vi "INIT R232 Seperate Mode.vi"(8 "error in (no error)":errorcluster, 11 "MC VISA resource in":refnum<visa-resource-name>="ASRL1::INSTR") -> (0 "MC error out":errorcluster, 1 "MC Init Complete":bool=TRUE, 3 "MC VISA resource  out":refnum<visa-resource-name>)   [LabVIEW 2009]
uses:
  <vilib>/Instr/_visa.llb/VISA Configure Serial Port (Instr).vi
panel:
  out "All Stop":bool
  out "Set Mode 3":bool
  in  "Mode command 3":string="^04 C0"
  out "Set Mode 2":bool
  in  "Mode command 2":string="^03 00"
  out "Set RS232 Control":bool
  out "Set Mode 1":bool
  in  "Mode command 1":string="^01 C4"
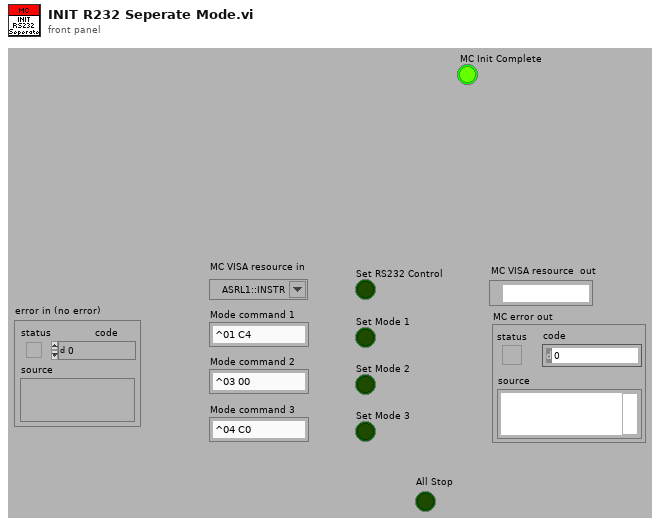
[diagram p1: front panel]
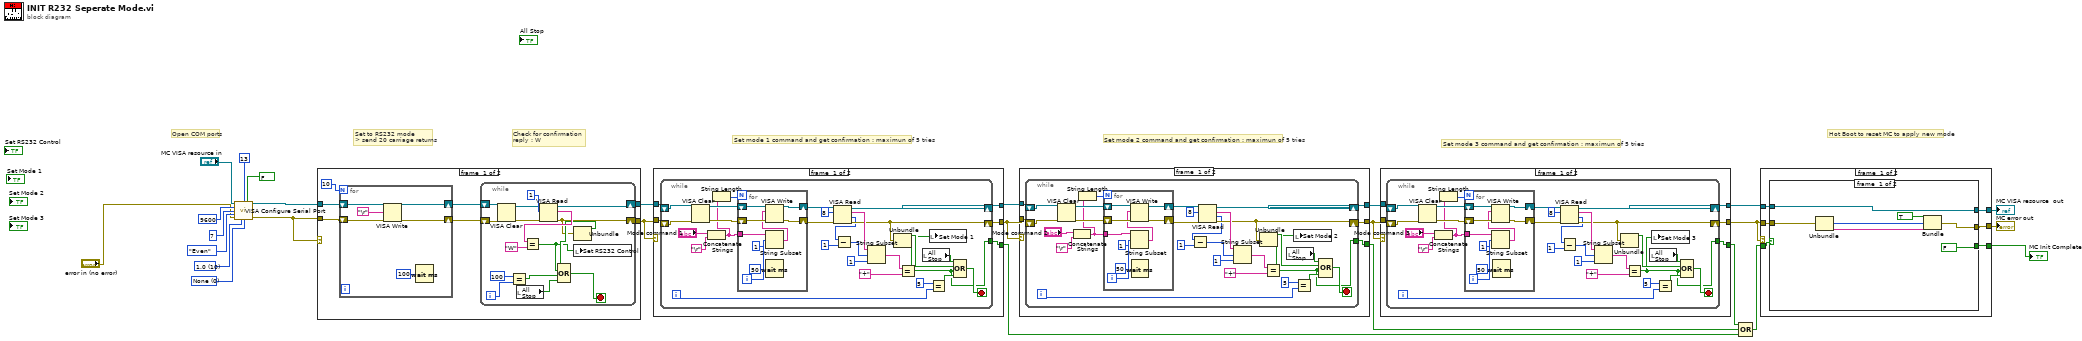
[diagram p0: block diagram]
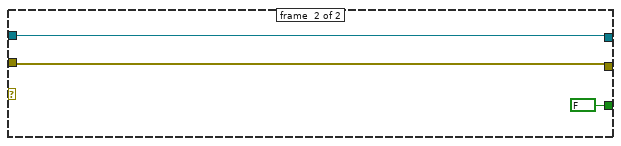
[diagram p2: hidden frame]
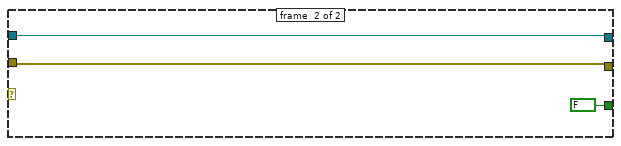
[diagram p3: hidden frame]
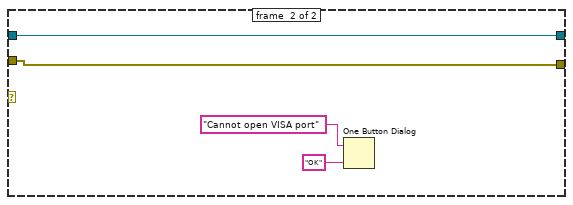
[diagram p4: hidden frame]
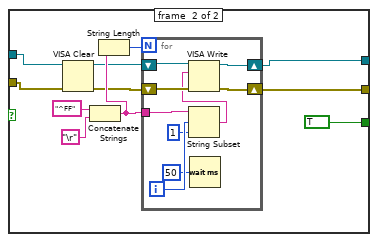
[diagram p5: hidden frame]
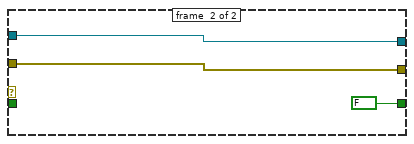
[diagram p6: hidden frame]
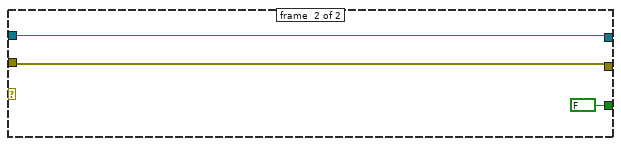
[diagram p7: hidden frame]
diagram:
  w22 = u16 0 items=["None", "XON/XOFF", "RTS/CTS", "XON/XOFF & RTS/CTS", "DTR/DSR", "XON/XOFF & DTR/DSR"] ("flow control (0:none)")
  w23 = u16 10 items=["1.0"=10, "1.5"=15, "2.0"=20] ("stop bits (10: 1 bit)")
  # "Set mode 3 command and get confirmation : maximun of 5 tries"
  # "Set mode 2 command and get confirmation : maximun of 5 tries"
  # "Hot Boot to reset MC to apply new mode"
  # "Check for confirmation\nreply : W"
  # "Set mode 1 command and get confirmation : maximun of 5 tries"
  # "Set to RS232 mode\n> send 20 carriage returns"
  # "Open COM ports"
  n1 = call-poly "VISA Configure Serial Port"("VISA resource name"="MC VISA resource in", "termination char\n(0xA = '\\n' = LF)"=u8 13 ("termination char\n(0xA = '\\n' = LF)"), "Enable Termination\nChar (T)"=FALSE ("Enable Termination\nChar (T)"), "baud rate (9600)"=u32 9600, "data bits (8)"=u16 7, "parity (0:none)"=enum16{"None", "Odd", "Even", "Mark", "Space"}."Even", "error in (no error)"="error in (no error)", "stop bits (10: 1 bit)"=w23, "flow control (0:none)"=w22) -> ("VISA resource name out"=w21:refnum<visa-resource-name>, "error out"=w17:errorcluster)  [unwired: 5 out]
  n2 = case shown="No Error" w17 {
    tunnel: w17 -> [w32 w58]
    tunnel: w21 -> [w31 w59]
    tunnel: [w30 w59] -> w20
    tunnel: [w27 w58] -> w18
    frame #0 {
      n3 = for {
        N: 10 -> [_]
        shift-right: [w52] -> w29
        shift-left: w32 -> [w55]
        shift-right: [w54] -> w28
        shift-left: w31 -> [w53]
        n4 = VISA Write(VISA resource name=w53, write buffer="\r", error in (no error)=w55) -> (VISA resource name out=w54:refnum<visa-resource-name>, error out=w52:errorcluster)  [unwired: 1 out]
        n5 = Wait (ms)(milliseconds to wait=u32 100) -> ()  [unwired: 1 out]
      }
      n6 = while {
        shift-right: [w45] -> w30
        shift-left: w28 -> [w46]
        shift-right: [w37] -> w27
        shift-left: w29 -> [w44]
        i -> [w41]
        stop <- w38 stop-if-true
        n7 = VISA Clear(VISA resource name=w46, error in (no error)=w44) -> (VISA resource name out=w43:refnum<visa-resource-name>, error out=w36:errorcluster)
        n8 = Equal?(x=100, y=w41) -> (x = y?=w39:bool)
        n9 = local read "All Stop"() -> (w34:bool)
        n10 = VISA Read(VISA resource name=w43, byte count=u32 1, error in (no error)=w36) -> (VISA resource name out=w45:refnum<visa-resource-name>, read buffer=w48:string, error out=w37:errorcluster)  [unwired: 1 out]
        n11 = Equal?(x=w48, y="W") -> (x = y?=w35:bool)
        n12 = Unbundle(w37) -> ("status"=w42:bool)  [unwired: 2 out]
        n13 = Compound Arithmetic op=OR(w42, w35, w39, w34) -> (w38:bool)
        n14 = local write "Set RS232 Control"(w35) -> ()
      }
    }
    frame #1 {
      n15 = One Button Dialog(message="Cannot open VISA port", button name ("OK")="OK") -> ()  [unwired: 1 out]
    }
  }
  n16 = case shown="No Error" w18 {
    tunnel: [w64 w103] -> w13
    tunnel: [w63 w102] -> w14
    tunnel: w20 -> [w62 w103]
    tunnel: w18 -> [w61 w102]
    tunnel: [w60 FALSE] -> w15
    frame #0 {
      n17 = while {
        shift-right: [w87] -> w64
        shift-left: w62 -> [w91]
        shift-right: [w76] -> w63
        shift-left: w61 -> [w90]
        tunnel: [w70] -> w60
        i -> [w73]
        stop <- w71 stop-if-true
        n18 = VISA Clear(VISA resource name=w91, error in (no error)=w90) -> (VISA resource name out=w84:refnum<visa-resource-name>, error out=w83:errorcluster)
        n19 = Concatenate Strings("Mode command 1", "\r") -> (w77:string)
        n20 = String Length(string=w77) -> (length=w78:i32)
        n21 = for {
          N: w78 -> [_]
          tunnel: w77 -> [w96]
          shift-right: [w100] -> w89
          shift-left: w83 -> [w97]
          shift-right: [w99] -> w88
          shift-left: w84 -> [w98]
          i -> [w95]
          n22 = String Subset(string=w96, offset (0)=w95, length (rest)=1 ("length (rest)")) -> (substring=w93:string)
          n23 = VISA Write(VISA resource name=w98, write buffer=w93, error in (no error)=w97) -> (VISA resource name out=w99:refnum<visa-resource-name>, error out=w100:errorcluster)  [unwired: 1 out]
          n24 = Wait (ms)(milliseconds to wait=u32 50) -> ()  [unwired: 1 out]
        }
        n25 = VISA Read(VISA resource name=w88, byte count=u32 8, error in (no error)=w89) -> (VISA resource name out=w87:refnum<visa-resource-name>, read buffer=w81:string, return count=w67:u32, error out=w76:errorcluster)
        n26 = Subtract(x=w67, y=u32 1) -> (x-y=w68:u32)
        n27 = String Subset(string=w81, offset (0)=w68, length (rest)=1 ("length (rest)")) -> (substring=w80:string)
        n28 = Unbundle(w76) -> ("status"=w72:bool)  [unwired: 2 out]
        n29 = Equal?(x=w80, y="+") -> (x = y?=w70:bool)
        n30 = local read "All Stop"() -> (w69:bool)
        n31 = local write "Set Mode 1"(w70) -> ()
        n32 = Equal?(x=5, y=w73) -> (x = y?=w74:bool)
        n33 = Compound Arithmetic op=OR(w69, w72, w70, w74) -> (w71:bool)
      }
    }
    frame #1 {
    }
  }
  n34 = case shown="No Error" w14 {
    tunnel: [w108 w147] -> w11
    tunnel: [w107 w146] -> w10
    tunnel: w13 -> [w106 w147]
    tunnel: w14 -> [w105 w146]
    tunnel: [w104 FALSE] -> w12
    frame #0 {
      n35 = while {
        shift-right: [w131] -> w108
        shift-left: w106 -> [w135]
        shift-right: [w120] -> w107
        shift-left: w105 -> [w134]
        tunnel: [w114] -> w104
        i -> [w117]
        stop <- w115 stop-if-true
        n36 = VISA Clear(VISA resource name=w135, error in (no error)=w134) -> (VISA resource name out=w128:refnum<visa-resource-name>, error out=w127:errorcluster)
        n37 = Concatenate Strings("Mode command 2", "\r") -> (w121:string)
        n38 = String Length(string=w121) -> (length=w122:i32)
        n39 = for {
          N: w122 -> [_]
          tunnel: w121 -> [w140]
          shift-right: [w144] -> w133
          shift-left: w127 -> [w141]
          shift-right: [w143] -> w132
          shift-left: w128 -> [w142]
          i -> [w139]
          n40 = String Subset(string=w140, offset (0)=w139, length (rest)=1 ("length (rest)")) -> (substring=w137:string)
          n41 = VISA Write(VISA resource name=w142, write buffer=w137, error in (no error)=w141) -> (VISA resource name out=w143:refnum<visa-resource-name>, error out=w144:errorcluster)  [unwired: 1 out]
          n42 = Wait (ms)(milliseconds to wait=u32 50) -> ()  [unwired: 1 out]
        }
        n43 = VISA Read(VISA resource name=w132, byte count=u32 8, error in (no error)=w133) -> (VISA resource name out=w131:refnum<visa-resource-name>, read buffer=w125:string, return count=w112:u32, error out=w120:errorcluster)
        n44 = Subtract(x=w112, y=u32 1) -> (x-y=w111:u32)
        n45 = String Subset(string=w125, offset (0)=w111, length (rest)=1 ("length (rest)")) -> (substring=w124:string)
        n46 = Unbundle(w120) -> ("status"=w116:bool)  [unwired: 2 out]
        n47 = Equal?(x=w124, y="+") -> (x = y?=w114:bool)
        n48 = local read "All Stop"() -> (w113:bool)
        n49 = local write "Set Mode 2"(w114) -> ()
        n50 = Equal?(x=5, y=w117) -> (x = y?=w118:bool)
        n51 = Compound Arithmetic op=OR(w113, w116, w114, w118) -> (w115:bool)
      }
    }
    frame #1 {
    }
  }
  n52 = case shown="No Error" w10 {
    tunnel: [w152 w191] -> w9
    tunnel: [w151 w190] -> w7
    tunnel: w11 -> [w150 w191]
    tunnel: w10 -> [w149 w190]
    tunnel: [w148 FALSE] -> w8
    frame #0 {
      n53 = while {
        shift-right: [w175] -> w152
        shift-left: w150 -> [w179]
        shift-right: [w164] -> w151
        shift-left: w149 -> [w178]
        tunnel: [w158] -> w148
        i -> [w161]
        stop <- w159 stop-if-true
        n54 = VISA Clear(VISA resource name=w179, error in (no error)=w178) -> (VISA resource name out=w172:refnum<visa-resource-name>, error out=w171:errorcluster)
        n55 = Concatenate Strings("Mode command 3", "\r") -> (w165:string)
        n56 = String Length(string=w165) -> (length=w166:i32)
        n57 = for {
          N: w166 -> [_]
          tunnel: w165 -> [w184]
          shift-right: [w188] -> w177
          shift-left: w171 -> [w185]
          shift-right: [w187] -> w176
          shift-left: w172 -> [w186]
          i -> [w183]
          n58 = String Subset(string=w184, offset (0)=w183, length (rest)=1 ("length (rest)")) -> (substring=w181:string)
          n59 = VISA Write(VISA resource name=w186, write buffer=w181, error in (no error)=w185) -> (VISA resource name out=w187:refnum<visa-resource-name>, error out=w188:errorcluster)  [unwired: 1 out]
          n60 = Wait (ms)(milliseconds to wait=u32 50) -> ()  [unwired: 1 out]
        }
        n61 = VISA Read(VISA resource name=w176, byte count=u32 8, error in (no error)=w177) -> (VISA resource name out=w175:refnum<visa-resource-name>, read buffer=w169:string, return count=w156:u32, error out=w164:errorcluster)
        n62 = Subtract(x=w156, y=u32 1) -> (x-y=w155:u32)
        n63 = String Subset(string=w169, offset (0)=w155, length (rest)=1 ("length (rest)")) -> (substring=w168:string)
        n64 = Unbundle(w164) -> ("status"=w160:bool)  [unwired: 2 out]
        n65 = Equal?(x=w168, y="+") -> (x = y?=w158:bool)
        n66 = local read "All Stop"() -> (w157:bool)
        n67 = local write "Set Mode 3"(w158) -> ()
        n68 = Equal?(x=5, y=w161) -> (x = y?=w162:bool)
        n69 = Compound Arithmetic op=OR(w157, w160, w158, w162) -> (w159:bool)
      }
    }
    frame #1 {
    }
  }
  n70 = Compound Arithmetic op=OR(w8, w12, w15) -> (w16:bool)
  n71 = case shown="No Error" w7 {
    tunnel: w7 -> [w197 w227]
    tunnel: w9 -> [w196 w226]
    tunnel: w16 -> [w193 _]
    tunnel: [w195 w227] -> w5
    tunnel: [w194 w226] -> w6
    tunnel: [w192 FALSE] -> w4
    frame #0 {
      n72 = case shown="False" w193 {
        tunnel: w197 -> [w203 w209]
        tunnel: w196 -> [w199 w208]
        tunnel: [w204 w207] -> w195
        tunnel: [w199 w206] -> w194
        tunnel: [FALSE TRUE] -> w192
        frame #0 {
          n73 = Unbundle(w203) -> ("code"=w201:i32, "source"=w202:string)  [unwired: 1 out]
          n74 = Bundle(TRUE, "code"=w201, "source"=w202) -> (w204:cluster{bool, "code":i32, "source":string})  [unwired: 1 out]
        }
        frame #1 {
          n75 = VISA Clear(VISA resource name=w208, error in (no error)=w209) -> (VISA resource name out=w212:refnum<visa-resource-name>, error out=w213:errorcluster)
          n76 = Concatenate Strings("^FF" ("string"), "\r") -> (w215:string)
          n77 = String Length(string=w215) -> (length=w214:i32)
          n78 = for {
            N: w214 -> [_]
            tunnel: w215 -> [w220]
            shift-right: [w224] -> w207
            shift-left: w213 -> [w221]
            shift-right: [w223] -> w206
            shift-left: w212 -> [w222]
            i -> [w219]
            n79 = String Subset(string=w220, offset (0)=w219, length (rest)=1 ("length (rest)")) -> (substring=w217:string)
            n80 = VISA Write(VISA resource name=w222, write buffer=w217, error in (no error)=w221) -> (VISA resource name out=w223:refnum<visa-resource-name>, error out=w224:errorcluster)  [unwired: 1 out]
            n81 = Wait (ms)(milliseconds to wait=u32 50) -> ()  [unwired: 1 out]
          }
        }
      }
    }
    frame #1 {
    }
  }
  "MC VISA resource  out" <- w6
  "MC error out" <- w5
  "MC Init Complete" <- w4
